vi "InitializeCOMInstrument.vi"(8 "error in (no error)":errorcluster, 11 "COM Instrument IN":refnum<visa-resource-name>="COM1") -> (0 "error out":errorcluster, 3 "COM Instrument OUT":refnum<visa-resource-name>)   [LabVIEW 2017, in "Thermal Shock.lvlib"]
uses:
  Thermal Shock.lvlib
  <vilib>/Instr/_visa.llb/VISA Configure Serial Port (Instr).vi
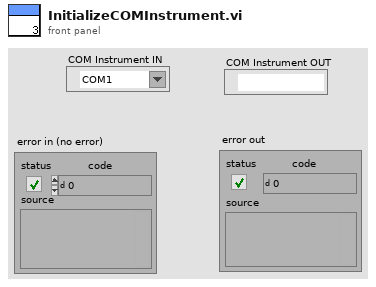
[diagram p1: front panel]
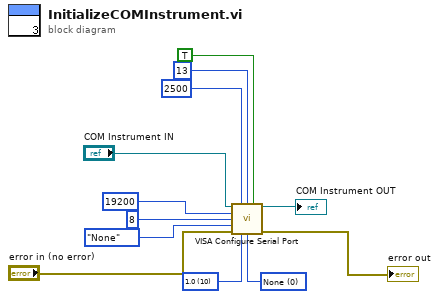
[diagram p0: block diagram]
diagram:
  w5 = u16 0 items=["None", "XON/XOFF", "RTS/CTS", "XON/XOFF & RTS/CTS", "DTR/DSR", "XON/XOFF & DTR/DSR"] ("flow control (0:none)")
  w7 = u16 10 items=["1.0"=10, "1.5"=15, "2.0"=20] ("stop bits (10: 1 bit)")
  n1 = call-poly "VISA Configure Serial Port"("VISA resource name"="COM Instrument IN", "timeout (10sec)"=2500, "termination char\n(0xA = '\\n' = LF)"=u8 13, "Enable Termination\nChar (T)"=TRUE, "baud rate (9600)"=19200, "data bits (8)"=u16 8, "parity (0:none)"=enum16{"None", "Odd", "Even", "Mark", "Space"}."None", "error in (no error)"="error in (no error)", "stop bits (10: 1 bit)"=w7, "flow control (0:none)"=w5) -> ("VISA resource name out"=→"COM Instrument OUT":refnum<visa-resource-name>, "error out"=→"error out":errorcluster)  [unwired: 4 in]
